vi "Read MessageInterface.vi"(11 "Proccess in":refnum<class "Proccess.lvclass">) -> (2 "MessageInterface":refnum<class "MessageInterface.lvclass">)   [LabVIEW 2019]
uses:
  Proccess.lvclass
  MessageInterface_class/MessageInterface.lvclass
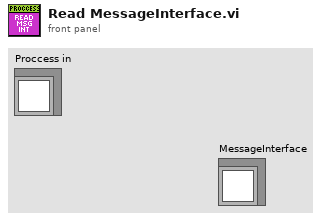
[diagram p1: front panel]
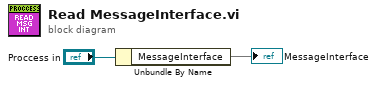
[diagram p0: block diagram]
diagram:
  n1 = Unbundle By Name("Proccess in") -> ("MessageInterface"=→"MessageInterface")
